vi "recycle_ccatch.vi"(8 "error in (no error)":errorcluster, 10 "s":bool) -> (0 "error out":errorcluster)   [LabVIEW 2019]
uses:
  servo state.ctl
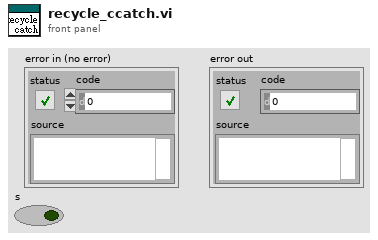
[diagram p1: front panel]
types:
  T1 = typedef "servo state.ctl" = enum16{"catch", "cam-1", "put", "side", "center", "side-2", "put-2"}
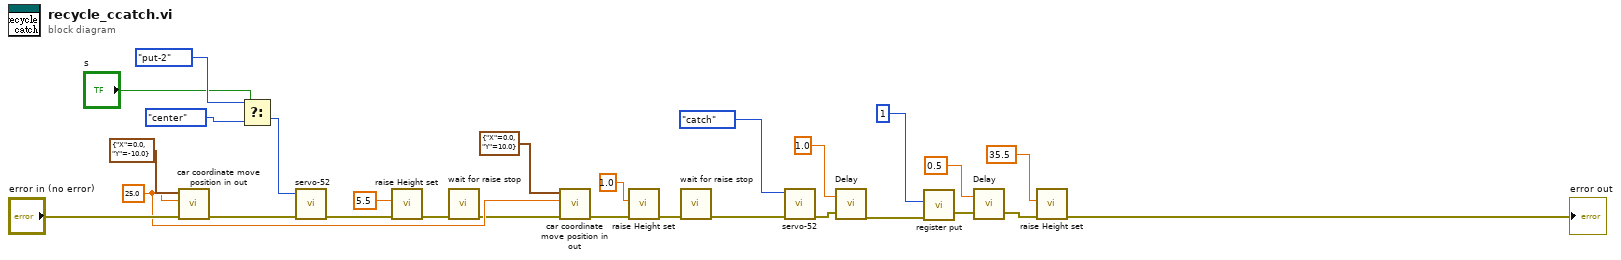
[diagram p0: block diagram]
diagram:
  w20 = 25.0 ("speed")
  n1 = call "car coordinate move position in out.vi"("error in (no error)"="error in (no error)", "speed"=w20, "move"=cluster{"X":dbl, "Y":dbl} {"X"=0.0, "Y"=-10.0}) -> ("error out"=w24:errorcluster)  [unwired: 7 in, 1 out]
  n2 = Select(t=servo_state."put-2", s="s", f=servo_state."center" ("Enum")) -> (s? t:f=w6:T1)
  n3 = call "servo-52.vi"("error in (no error)"=w24, "Enum"=w6) -> ("error out"=w25:errorcluster)  [unwired: 9 in]
  n4 = call "raise Height set.vi"("error in (no error)"=w25, "Height_cm"=5.5) -> ("error out"=w26:errorcluster)  [unwired: 9 in]
  n5 = call "wait for raise stop.vi"("Error In"=w26) -> ("Error Out"=w19:errorcluster)  [unwired: 10 in]
  n6 = call "car coordinate move position in out.vi"("error in (no error)"=w19, "speed"=w20, "move"=cluster{"X":dbl, "Y":dbl} {"X"=0.0, "Y"=10.0}) -> ("error out"=w18:errorcluster)  [unwired: 7 in, 1 out]
  n7 = call "raise Height set.vi"("error in (no error)"=w18, "Height_cm"=1.0) -> ("error out"=w16:errorcluster)  [unwired: 9 in]
  n8 = call "wait for raise stop.vi"("Error In"=w16) -> ("Error Out"=w15:errorcluster)  [unwired: 10 in]
  n9 = call "servo-52.vi"("error in (no error)"=w15, "Enum"=servo_state."catch") -> ("error out"=w13:errorcluster)  [unwired: 9 in]
  n10 = call "Delay.vi"("error in (no error)"=w13, "Delay Time (s)"=1.0) -> ("error out"=w12:errorcluster)  [unwired: 1 in]
  n11 = call "register put.vi"("error in (no error)"=w12, "register address"=1) -> ("error out"=w9:errorcluster)  [unwired: 9 in]
  n12 = call "Delay.vi"("error in (no error)"=w9, "Delay Time (s)"=0.5) -> ("error out"=w8:errorcluster)  [unwired: 1 in]
  n13 = call "raise Height set.vi"("error in (no error)"=w8, "Height_cm"=35.5) -> ("error out"=→"error out":errorcluster)  [unwired: 9 in]
